vi "test-numerical-jacobian.vi"() -> (3 "ALL Tests Passed":bool)   [LabVIEW 2019]
uses:
  <vilib>/Analysis/Matrix/Datatypes/RealMatrix.ctl
  <vilib>/Rock Robotics/WPI/ThirdParty/JAS_Junk/TrajLib/MatBuilder_Create.vi
  <vilib>/Rock Robotics/WPI/ThirdParty/JAS_Junk/TrajLib/Trajectory_Library.lvlib
  <vilib>/Analysis/Matrix/NI_Matrix.lvlib
panel:
  out "TEst Passed 0":bool
  out "TEst Passed 1":bool
  out "D":T1
  out "Error 1":bool
  out "Result 1":T1
  out "A":T1
  out "Error 0":bool
  out "Result 0":T1
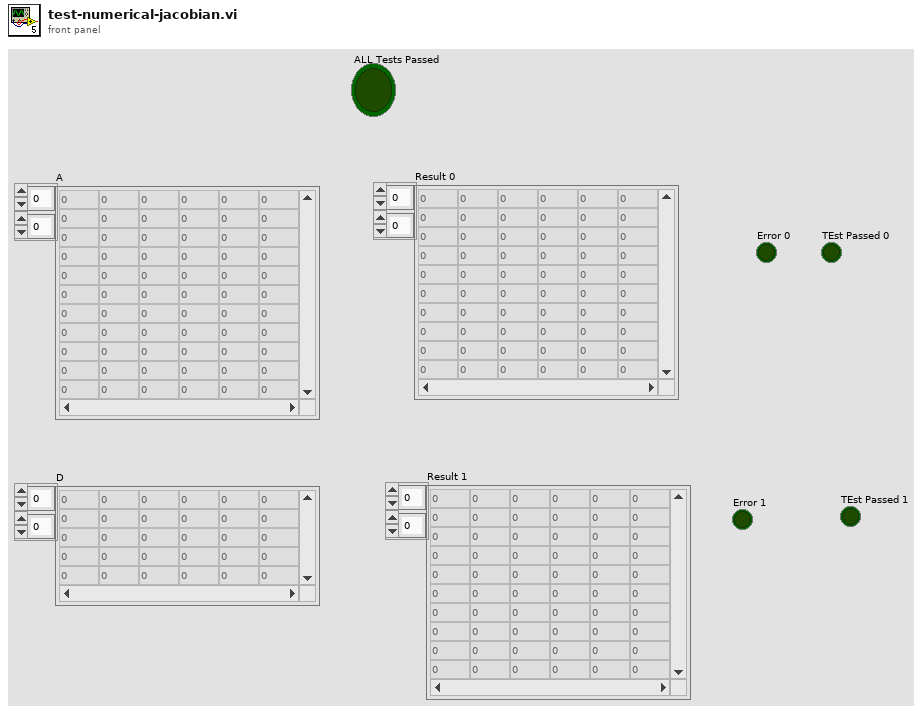
[diagram p1: front panel]
types:
  T1 = typedef "NI_Matrix.lvlib/RealMatrix.ctl" = dbl[][]
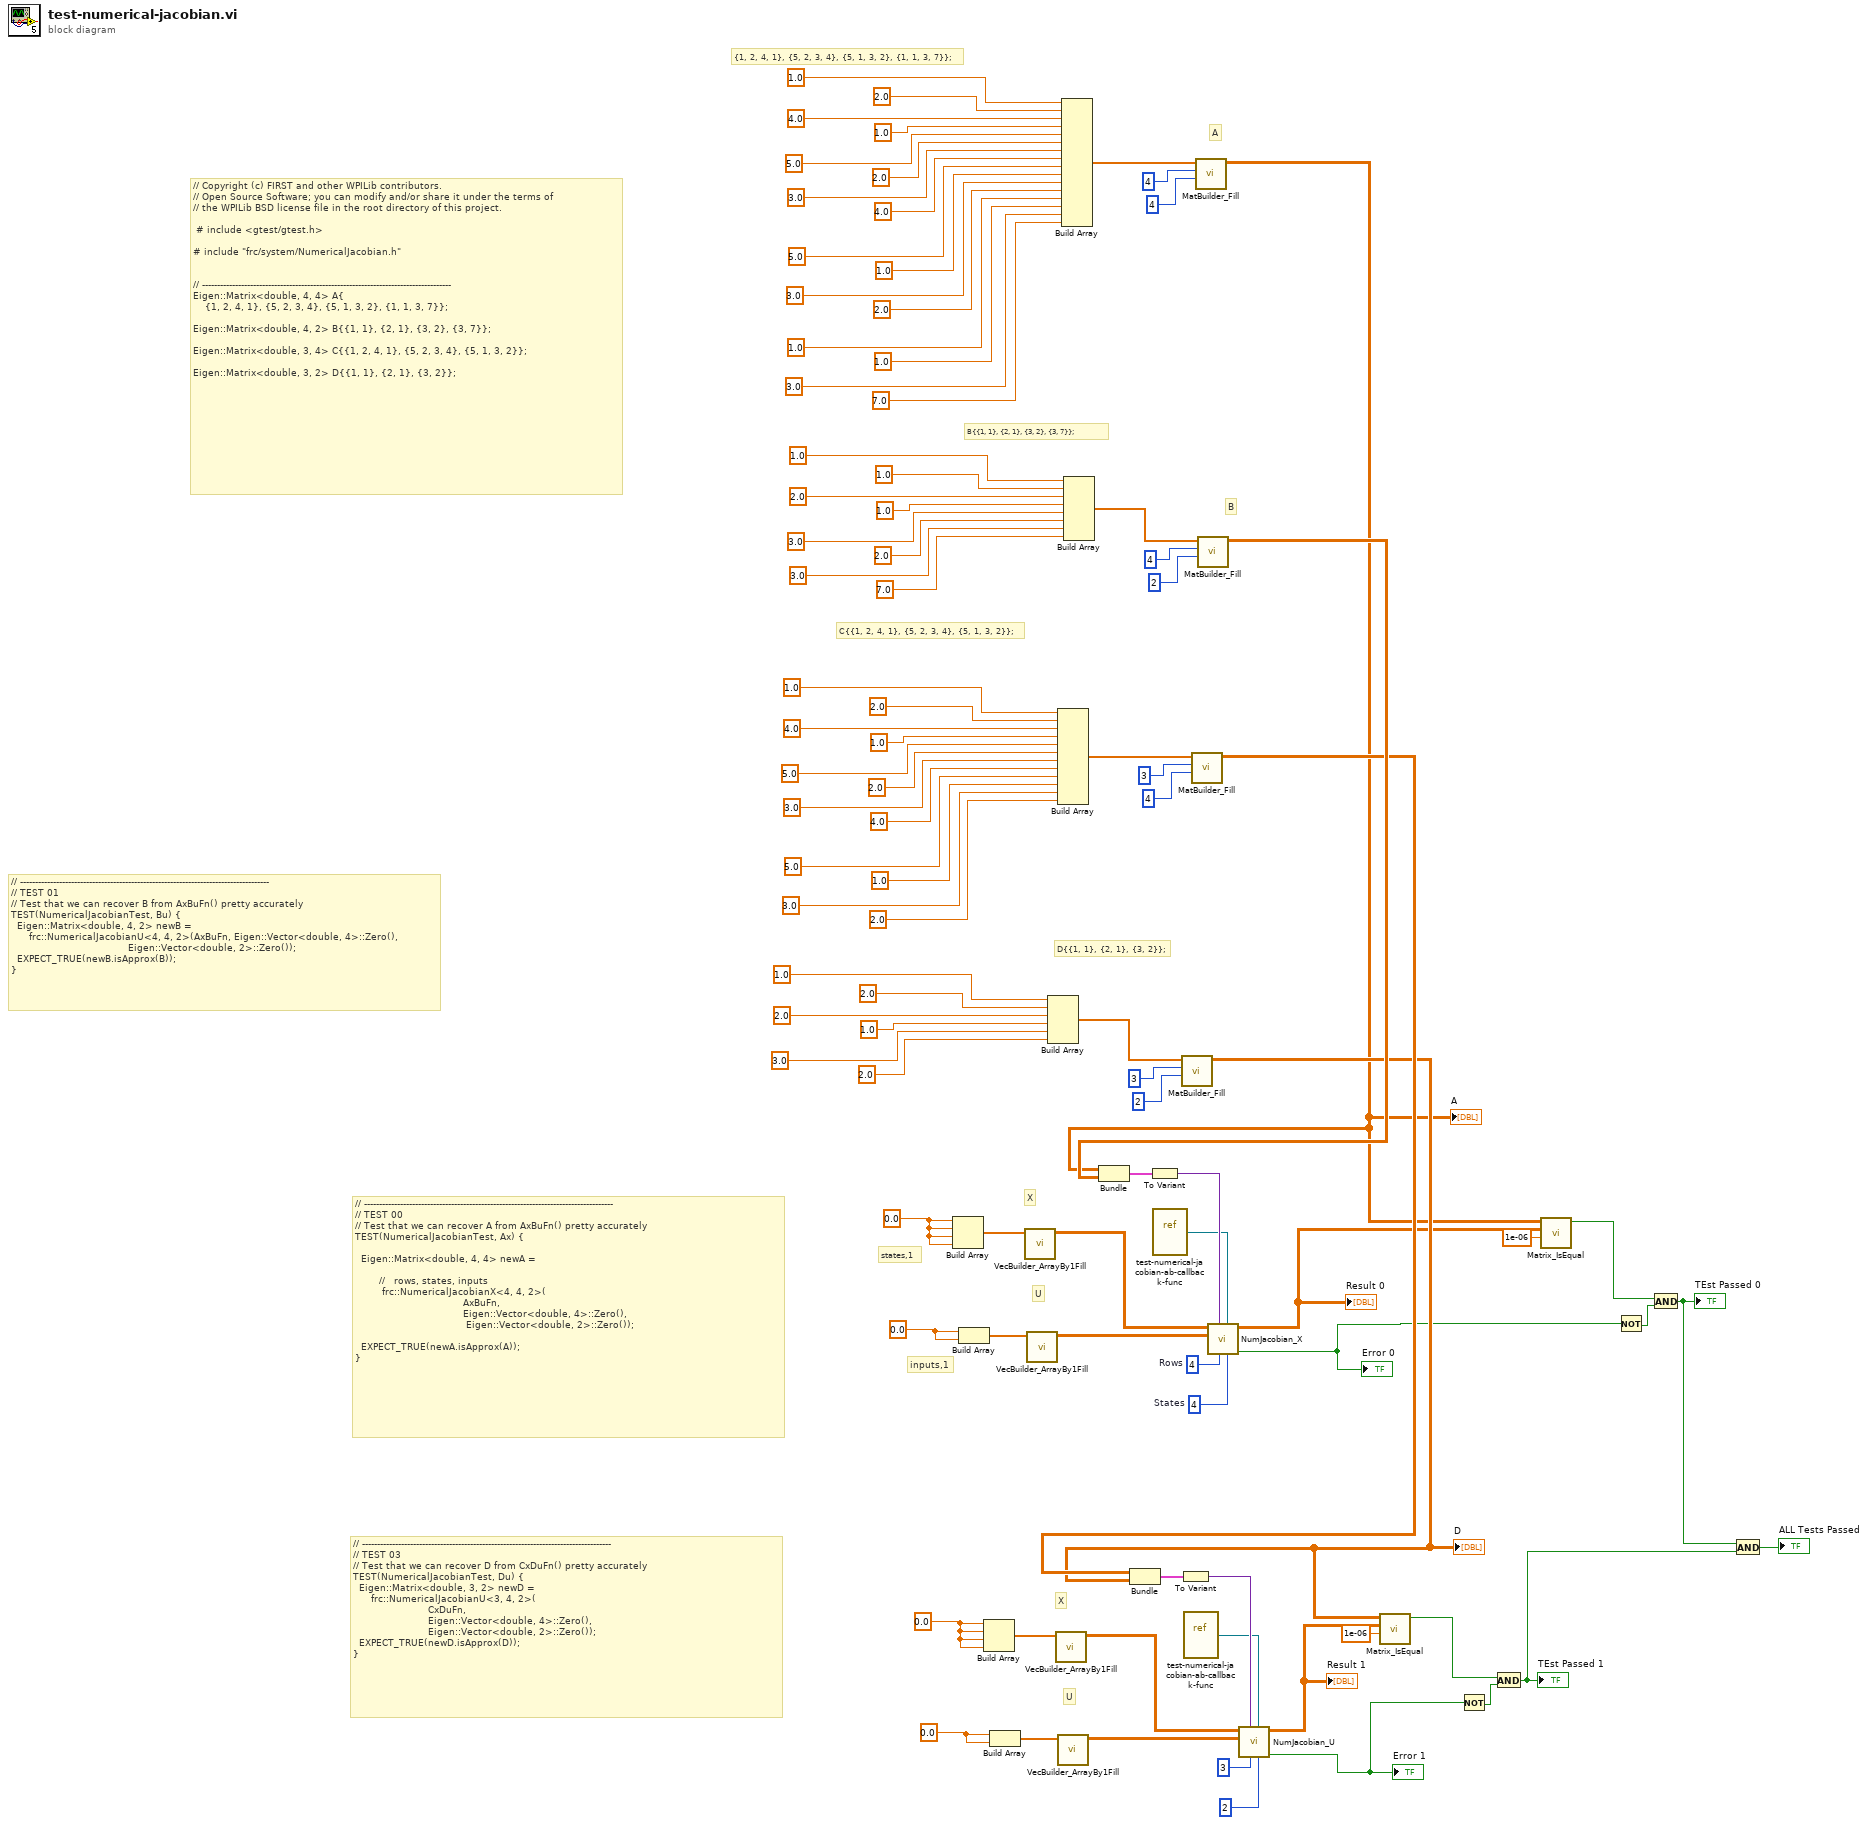
[diagram p0: block diagram]
diagram:
  w24 = 0.0 ("element")
  w26 = 0.0 ("element")
  w28 = 4  # States
  w29 = 4  # Rows
  w36 = 0.0 ("element")
  w38 = 0.0 ("element")
  # "inputs,1"
  # "states,1"
  # "U"
  # "X"
  # "B"
  # "A"
  # "U"
  # "X"
  # "D{{1, 1}, {2, 1}, {3, 2}};"
  # "C{{1, 2, 4, 1}, {5, 2, 3, 4}, {5, 1, 3, 2}};"
  # "B{{1, 1}, {2, 1}, {3, 2}, {3, 7}};"
  # "{1, 2, 4, 1}, {5, 2, 3, 4}, {5, 1, 3, 2}, {1, 1, 3, 7}};"
  # "// -----------------------------------------------------------------------------------\n// TEST 00\n// Test that we can recover A from AxBuFn() pretty accurately\nTEST(NumericalJacobianTest, Ax) {\n\n  Eigen::Matrix<double, 4, 4> newA =\n     \n        //   rows, states, inputs \n         frc::NumericalJacobianX<4, 4, 2>(\n                                    AxBuFn, \n                                    Eigen::Vector<double, 4>::Zero(),\n                                     Eigen::Vector<double, 2>::Zero());\n\n  EXPECT_TRUE(newA.isApprox(A));\n}"
  # "// -----------------------------------------------------------------------------------\n// TEST 01\n// Test that we can recover B from AxBuFn() pretty accurately\nTEST(NumericalJacobianTest, Bu) {\n  Eigen::Matrix<double, 4, 2> newB =\n      frc::NumericalJacobianU<4, 4, 2>(AxBuFn, Eigen::Vector<double, 4>::Zero(),\n                                       Eigen::Vector<double, 2>::Zero());\n  EXPECT_TRUE(newB.isApprox(B));\n}"
  # "// -----------------------------------------------------------------------------------\n// TEST 03\n// Test that we can recover D from CxDuFn() pretty accurately\nTEST(NumericalJacobianTest, Du) {\n  Eigen::Matrix<double, 3, 2> newD =\n      frc::NumericalJacobianU<3, 4, 2>(\n                         CxDuFn, \n                         Eigen::Vector<double, 4>::Zero(),\n                         Eigen::Vector<double, 2>::Zero());\n  EXPECT_TRUE(newD.isApprox(D));\n}"
  # "// Copyright (c) FIRST and other WPILib contributors.\n// Open Source Software; you can modify and/or share it under the terms of\n// the WPILib BSD license file in the root directory of this project.\n\n # include <gtest/gtest.h>\n\n# include \"frc/system/NumericalJacobian.h\"\n\n\n// -----------------------------------------------------------------------------------\nEigen::Matrix<double, 4, 4> A{\n    {1, 2, 4, 1}, {5, 2, 3, 4}, {5, 1, 3, 2}, {1, 1, 3, 7}};\n\nEigen::Matrix<double, 4, 2> B{{1, 1}, {2, 1}, {3, 2}, {3, 7}};\n\nEigen::Matrix<double, 3, 4> C{{1, 2, 4, 1}, {5, 2, 3, 4}, {5, 1, 3, 2}};\n\nEigen::Matrix<double, 3, 2> D{{1, 1}, {2, 1}, {3, 2}};"
  n1 = Build Array(w38, w38, w38, w38) -> (w39:dbl[])
  n2 = Build Array(w36, w36) -> (w37:dbl[])
  n3 = Build Array(w26, w26, w26, w26) -> (w27:dbl[])
  n4 = Build Array(w24, w24) -> (w25:dbl[])
  n5 = call <vilib>:"VecBuilder_ArrayBy1Fill.vi"("R Array"=w39) -> ("Output Vector"=w35:T1)  [unwired: 10 in]
  n6 = call <vilib>:"VecBuilder_ArrayBy1Fill.vi"("R Array"=w37) -> ("Output Vector"=w34:T1)  [unwired: 10 in]
  n7 = Build Array(1.0 ("element"), 2.0 ("element"), 2.0 ("element"), 1.0 ("element"), 3.0 ("element"), 2.0 ("element")) -> (w48:dbl[])
  n8 = call <vilib>:"VecBuilder_ArrayBy1Fill.vi"("R Array"=w27) -> ("Output Vector"=w23:T1)  [unwired: 10 in]
  n9 = Build Array(1.0 ("element"), 2.0 ("element"), 4.0 ("element"), 1.0 ("element"), 5.0 ("element"), 2.0 ("element"), 3.0 ("element"), 4.0 ("element"), 5.0 ("element"), 1.0 ("element"), 3.0 ("element"), 2.0 ("element")) -> (w63:dbl[])
  n10 = call <vilib>:"VecBuilder_ArrayBy1Fill.vi"("R Array"=w25) -> ("Output Vector"=w22:T1)  [unwired: 10 in]
  n11 = Build Array(1.0 ("element"), 2.0 ("element"), 4.0 ("element"), 1.0 ("element"), 5.0 ("element"), 2.0 ("element"), 3.0 ("element"), 4.0 ("element"), 5.0 ("element"), 1.0 ("element"), 3.0 ("element"), 2.0 ("element"), 1.0 ("element"), 1.0 ("element"), 3.0 ("element"), 7.0 ("element")) -> (w93:dbl[])
  n12 = Build Array(1.0 ("element"), 1.0 ("element"), 2.0 ("element"), 1.0 ("element"), 3.0 ("element"), 2.0 ("element"), 3.0 ("element"), 7.0 ("element")) -> (w74:dbl[])
  n13 = vi-ref "test-numerical-jacobian-ab-callback-func.vi"() -> (w30:refnum<vi>)
  n14 = call <vilib>:"MatBuilder_Fill.vi"("Columns"=2, "Rows"=3, "Value List"=w48) -> ("output matrix"=w15:T1)  [unwired: 8 in]
  "D" <- w15
  n15 = vi-ref "test-numerical-jacobian-ab-callback-func.vi"() -> (w19:refnum<vi>)
  n16 = call <vilib>:"MatBuilder_Fill.vi"("Columns"=4, "Rows"=3, "Value List"=w63) -> ("output matrix"=w16:T1)  [unwired: 8 in]
  n17 = Bundle("output matrix"=w16, "output matrix"=w15) -> (w21:cluster{"output matrix":T1, "output matrix":T1})  [unwired: 1 in]
  n18 = To Variant(anything=w21) -> (Variant=w20:variant)
  n19 = call <vilib>:"MatBuilder_Fill.vi"("Columns"=4, "Rows"=4, "Value List"=w93) -> ("output matrix"=w6:T1)  [unwired: 8 in]
  "A" <- w6
  n20 = call <vilib>:"MatBuilder_Fill.vi"("Columns"=2, "Rows"=4, "Value List"=w74) -> ("output matrix"=w33:T1)  [unwired: 8 in]
  n21 = Bundle("output matrix"=w6, "output matrix"=w33) -> (w32:cluster{"output matrix":T1, "output matrix":T1})  [unwired: 1 in]
  n22 = To Variant(anything=w32) -> (Variant=w31:variant)
  n23 = call <vilib>:"NumJacobian_X.vi"("States"=w28, "F_FUNC"=w30, "Rows"=w29, "ExtraPassedData"=w31, "U"=w34, "X"=w35) -> ("Error"=w4:bool, "Result"=w5:T1)  [unwired: 4 in]
  "Result 0" <- w5
  "Error 0" <- w4
  n24 = call <vilib>:"NumJacobian_U.vi"("Inputs"=2 ("States"), "F_FUNC"=w19, "Rows"=3, "ExtraPassedData"=w20, "U"=w22, "X"=w23) -> ("Error"=w11:bool, "Result"=w14:T1)  [unwired: 4 in]
  "Result 1" <- w14
  "Error 1" <- w11
  n25 = call <vilib>:"Matrix_IsEqual.vi"("Tolerance"=1e-06, "other"=w14, "input matrix"=w15) -> ("Equal"=w12:bool)  [unwired: 8 in]
  n26 = Not(x=w11) -> (.not. x?=w10:bool)
  n27 = And(x=w12, y=w10) -> (x .and. y?=w1:bool)
  "TEst Passed 1" <- w1
  n28 = call <vilib>:"Matrix_IsEqual.vi"("Tolerance"=1e-06, "other"=w5, "input matrix"=w6) -> ("Equal"=w8:bool)  [unwired: 8 in]
  n29 = Not(x=w4) -> (.not. x?=w7:bool)
  n30 = And(x=w8, y=w7) -> (x .and. y?=w2:bool)
  "TEst Passed 0" <- w2
  n31 = And(x=w2, y=w1) -> (x .and. y?=→"ALL Tests Passed":bool)
